vi "MiniBatchDictionaryLearning.vi"(8 "error in":errorcluster) -> (0 "error out":errorcluster, 3 "out":refnum<class "MiniBatchDictionaryLearning.lvclass">)   [LabVIEW 2020]
doc: "Mini-batch dictionary learning\n\n Finds a dictionary (a set of atoms) that can best be used to represent data\n using a sparse code.\n\n Solves the optimization problem::\n\n (U^*,V^*) = argmin 0.5 || X - U V ||_2^2 + alpha * || U ||_1\n (U,V)\n with || V_k ||_2 = 1 for all 0 <= k < n_components\n\n Read more in the :ref:`User Guide <DictionaryLearning>`.\n\n Parameters\n ----------\n n_components : int, default=None\n Number of dictionary elements to extract.\n\n alpha : float, default=1\n Sparsity controlling parameter.\n\n n_iter : int, default=1000\n Total number of iterations to perform.\n\n fit_algorithm : {'lars', 'cd'}, default='lars'\n The algorithm used:\n\n - `'lars'`: uses the least angle regression method to solve the lasso\n problem (`linear_model.lars_path`)\n - `'cd'`: uses the coordinate descent method to compute the\n Lasso solution (`linear_model.Lasso`). Lars will be faster if\n the estimated components are sparse.\n\n n_jobs : int, default=None\n Number of parallel jobs to run.\n ``None`` means 1 unless in a :obj:`joblib.parallel_backend` context.\n ``-1`` means using all processors. See :term:`Glossary <n_jobs>`\n for more details.\n\n batch_size : int, default=3\n Number of samples in each mini-batch.\n\n shuffle : bool, default=True\n Whether to shuffle the samples before forming batches.\n\n dict_init : ndarray of shape (n_components, n_features), default=None\n initial value of the dictionary for warm restart scenarios\n\n transform_algorithm : {'lasso_lars', 'lasso_cd', 'lars', 'omp', 'threshold'}, default='omp'\n Algorithm used to transform the data:\n\n - `'lars'`: uses the least angle regression method\n (`linear_model.lars_path`);\n - `'lasso_lars'`: uses Lars to compute the Lasso solution.\n - `'lasso_cd'`: uses the coordinate descent method to compute the\n Lasso solution (`linear_model.Lasso`). `'lasso_lars'` will be faster\n if the estimated components are sparse.\n - `'omp'`: uses orthogonal matching pursuit to estimate the sparse\n solution.\n - `'threshold'`: squashes to zero all coefficients less than alpha from\n the projection ``dictionary * X'``.\n\n transform_n_nonzero_coefs : int, default=None\n Number of nonzero coefficients to target in each column of the\n solution. This is only used by `algorithm='lars'` and `algorithm='omp'`\n and is overridden by `alpha` in the `omp` case. If `None`, then\n `transform_n_nonzero_coefs=int(n_features / 10)`.\n\n transform_alpha : float, default=None\n If `algorithm='lasso_lars'` or `algorithm='lasso_cd'`, `alpha` is the\n penalty applied to the L1 norm.\n If `algorithm='threshold'`, `alpha` is the absolute value of the\n threshold below which coefficients will be squashed to zero.\n If `algorithm='omp'`, `alpha` is the tolerance parameter: the value of\n the reconstruction error targeted. In this case, it overrides\n `n_nonzero_coefs`.\n If `None`, default to 1.\n\n verbose : bool, default=False\n To control the verbosity of the procedure.\n\n split_sign : bool, default=False\n Whether to split the sparse feature vector into the concatenation of\n its negative part and its positive part. This can improve the\n performance of downstream classifiers.\n\n random_state : int, RandomState instance or None, default=None\n Used for initializing the dictionary when ``dict_init`` is not\n specified, randomly shuffling the data when ``shuffle`` is set to\n ``True``, and updating the dictionary. Pass an int for reproducible\n results across multiple function calls.\n See :term:`Glossary <random_state>`.\n\n positive_code : bool, default=False\n Whether to enforce positivity when finding the code.\n\n .. versionadded:: 0.20\n\n positive_dict : bool, default=False\n Whether to enforce positivity when finding the dictionary.\n\n .. versionadded:: 0.20\n\n transform_max_iter : int, default=1000\n Maximum number of iterations to perform if `algorithm='lasso_cd'` or\n `'lasso_lars'`.\n\n .. versionadded:: 0.22\n\n Attributes\n ----------\n components_ : ndarray of shape (n_components, n_features)\n Components extracted from the data.\n\n inner_stats_ : tuple of (A, B) ndarrays\n Internal sufficient statistics that are kept by the algorithm.\n Keeping them is useful in online settings, to avoid losing the\n history of the evolution, but they shouldn't have any use for the\n end user.\n `A` `(n_components, n_components)` is the dictionary covariance matrix.\n `B` `(n_features, n_components)` is the data approximation matrix.\n\n n_iter_ : int\n Number of iterations run.\n\n iter_offset_ : int\n The number of iteration on data batches that has been\n performed before.\n\n random_state_ : RandomState instance\n RandomState instance that is generated either from a seed, the random\n number generattor or by `np.random`.\n\n \nAvailable methods:\nFit\nFit Transform\nTransform\nGet Attributes\nGet Params\nSet Params"
uses:
  MiniBatchDictionaryLearning.lvclass
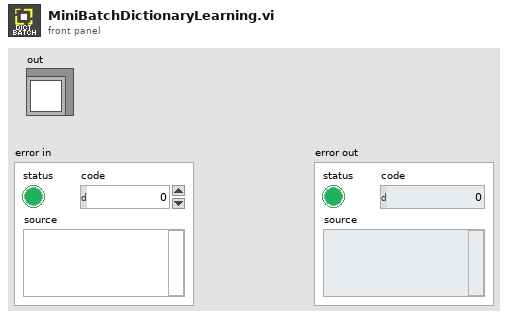
[diagram p1: front panel]
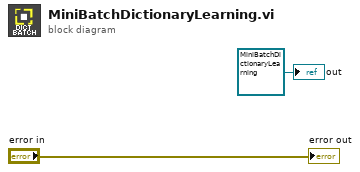
[diagram p0: block diagram]
diagram:
  "out" <- refnum<class "MiniBatchDictionaryLearning.lvclass"> refnum ("model")
  "error out" <- "error in"
